vi "CleanUp.vi"(0 "object in":refnum<class "NI-XNET.lvclass">, 11 "error in (no error)":errorcluster) -> (4 "object out":refnum<class "NI-XNET.lvclass">, 15 "error out":errorcluster)   [LabVIEW 2023, in "HardwareAbstractionLayer_LVOOP.lvlib" / "CAN HAL Lib.lvlib" / "NI-XNET.lvclass"]
uses:
  NI-XNET.lvclass
  NI-XNET.lvclass/NI-XNET.ctl
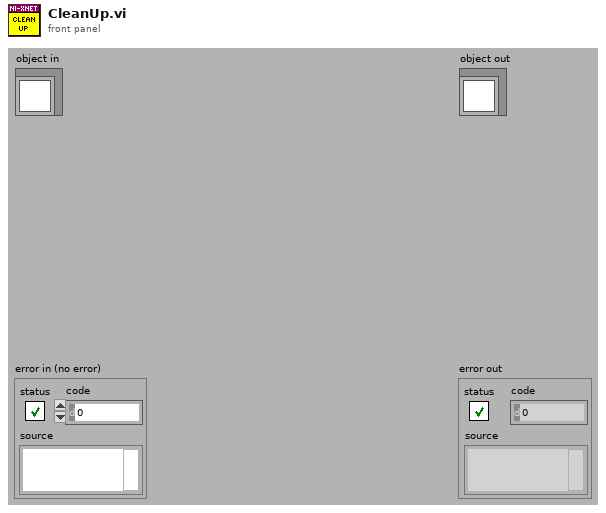
[diagram p1: front panel]
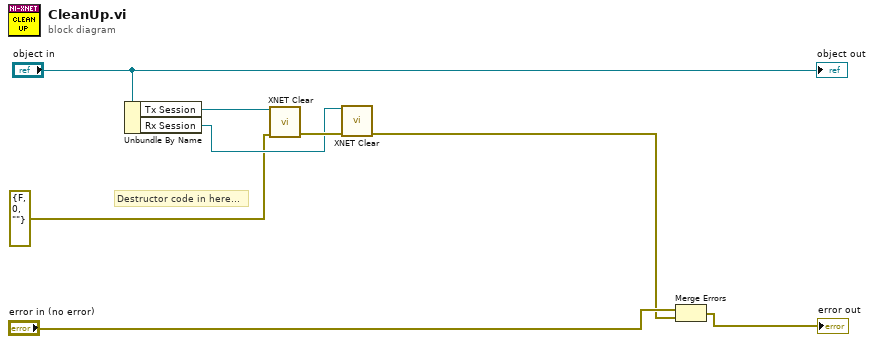
[diagram p0: block diagram]
diagram:
  # "Destructor code in here..."
  n1 = Unbundle By Name("object in") -> ("Tx Session"=w7:refnum<k21>, "Rx Session"=w5:refnum<k21>)
  n2 = call <vilib>:"XNET Clear.vi"("session in"=w7, "error in (no error)"=errorcluster {"status"=FALSE, "code"=0, "source"=""}) -> ("error out"=w6:errorcluster)  [unwired: 13 in]
  n3 = call <vilib>:"XNET Clear.vi"("session in"=w5, "error in (no error)"=w6) -> ("error out"=w3:errorcluster)  [unwired: 13 in]
  n4 = Merge Errors("error in (no error)", w3) -> (→"error out":errorcluster)
  "object out" <- "object in"
